vi "阈值图像分割.vi"() -> ()   [LabVIEW 2018]
doc: "This example shows how to open, read, and display an AVI file in NI Vision. The VI reads the frames per second property and plays the images back at the rate specified by the AVI file."
uses:
  <vilib>/Utility/file.llb/Read Delimited Spreadsheet (DBL).vi
  <vilib>/Utility/file.llb/Write Delimited Spreadsheet (I64).vi
  <vilib>/vision/NI_Vision_Development_Module.lvlib
panel:
  in  "清除叠加火焰":bool
  in  "保存":bool
  out "像素当量单位":string
  out "像素当量":string
  out "帧数据":T1
  in  "保存按钮":bool
  out "叠加像素源":u8[][](array[numeric])
  out "总像素":dbl
  in  "暂停按钮":bool
  out "火焰帧数":string
  out "叠加实际":string
  out "单帧实际":string
  out "叠加像素":string
  out "单帧像素":string
  out "导入像素当量":bool
  in  "单帧回看":bool
  out "叠加部分":string
  out "单帧部分":string
  in  "火焰详细参数":bool
  in  "返回主界面":bool
  out "a直方图":dynamicdata(graph) caption="A直方图"
  out "L直方图":dynamicdata(graph)
  in  "b":cluster{i32, i32}(slide)={-21, 6} scale=-100.0..100.0
  in  "a":cluster{i32, i32}(slide)={-21, -7} scale=-100.0..100.0
  in  "L":cluster{i32, i32}(slide)={81, 99} scale=0.0..100.0
  out "图形处理后":T2(plugin-control)
  out "单幅画面":T2(plugin-control) caption="单帧画面"
  in  "帧数计数":i32(slide) max=25 scale=0.0..25.0
  in  "Stop":bool
  out "Threshold Image":T2(plugin-control) caption="原图"
  out "叠加画面":T2(plugin-control)
  out "b直方图":dynamicdata(graph) caption="B直方图"
  # "基于Lab颜色空间的炮口火焰阈值分割"
  # "火焰参数"
  # "Lab颜色直方图&阈值选择"
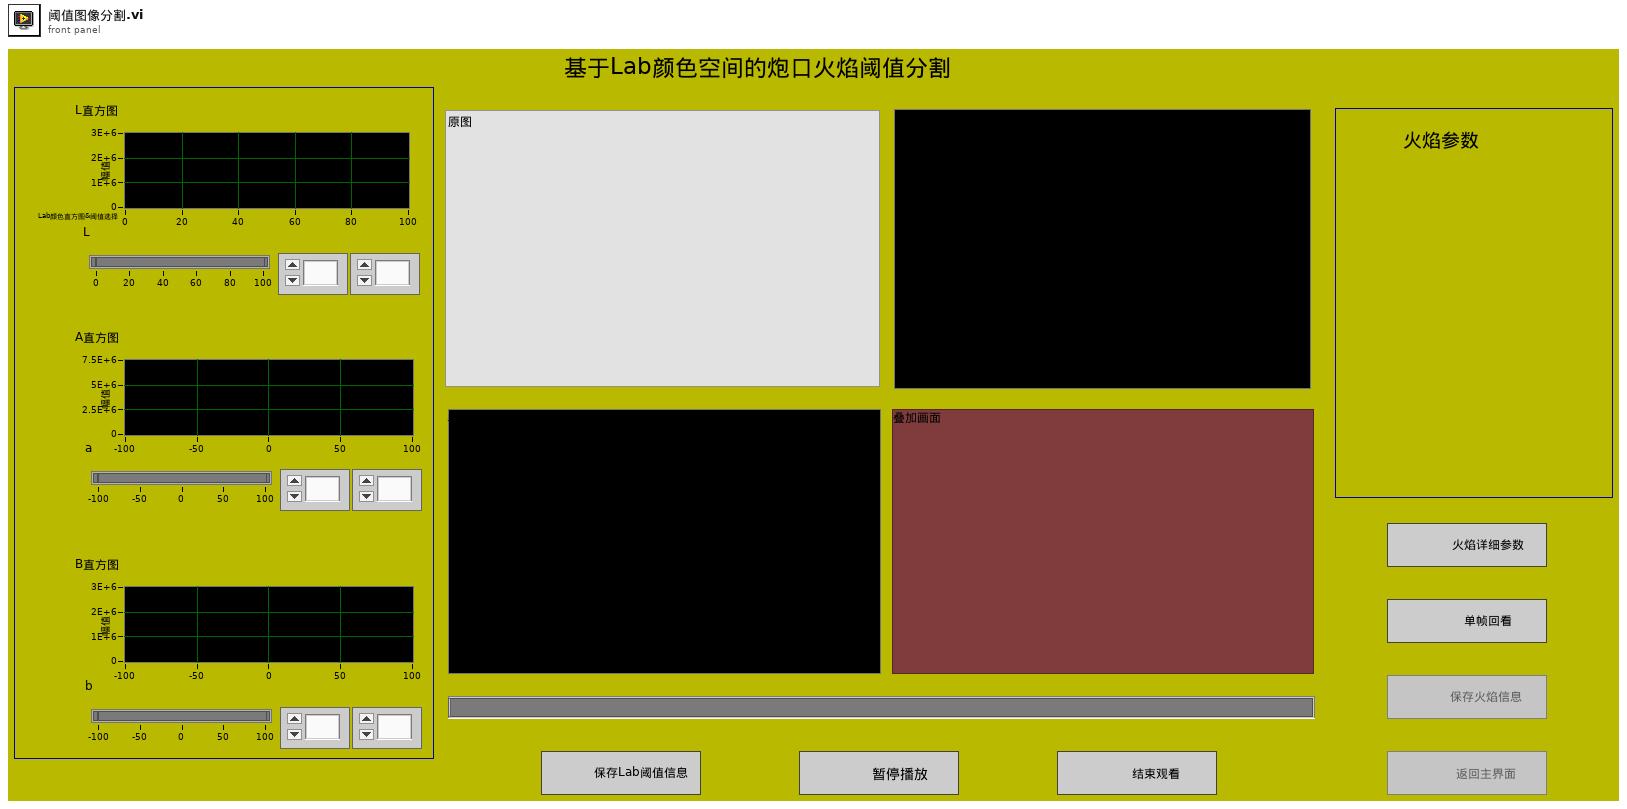
[diagram p1: front panel]
types:
  T1 = cluster{"Width":u32, "Height":u32, "Frames Per Second":u32, "Codec":string, "Has Data":bool}
  T2 = typedef "IMAQ Image.ctl" = refnum<image>
  T3 = enum8{"Enabled", "Disabled", "Disabled and Grayed Out"}
  T4 = typedef "Image Type" = u32
  T5 = enum32{"Invalid", "Standard", "Closed", "Hidden", "Minimized", "Maximized"}
  T6 = typedef "IMAQ AVI2 Refnum.ctl" = refnum<k20>
  T7 = cluster{"X Size":i32, "Y Size":i32, "% Tolerance":i32}
  T8 = typedef "ROI Descriptor" = cluster{"Global Rectangle":i32[], "Contours":cluster{"ID":enum32{"External", "Internal"}, "Type":u32, "Coordinates":i32[]}[]}
  T9 = cluster{"Area":dbl, "Number of Holes":dbl, "Bounding Rect":cluster{"Left":dbl, "Top":dbl, "Right":dbl, "Bottom":dbl}, "Center of Mass":cluster{"X":dbl, "Y":dbl}, "Orientation":dbl, "Dimensions":cluster{"Width":dbl, "Height":dbl}}[]
  T10 = cluster{"Particle Reports (Pixels)[0]":cluster{"Area":dbl, "Number of Holes":dbl, "Bounding Rect":cluster{"Left":dbl, "Top":dbl, "Right":dbl, "Bottom":dbl}, "Center of Mass":cluster{"X":dbl, "Y":dbl}, "Orientation":dbl, "Dimensions":cluster{"Width":dbl, "Height":dbl}}, "Particle Reports (Pixels)[1]":cluster{"Area":dbl, "Number of Holes":dbl, "Bounding Rect":cluster{"Left":dbl, "Top":dbl, "Right":dbl, "Bottom":dbl}, "Center of Mass":cluster{"X":dbl, "Y":dbl}, "Orientation":dbl, "Dimensions":cluster{"Width":dbl, "Height":dbl}}, "Particle Reports (Pixels)[2]":cluster{"Area":dbl, "Number of Holes":dbl, "Bounding Rect":cluster{"Left":dbl, "Top":dbl, "Right":dbl, "Bottom":dbl}, "Center of Mass":cluster{"X":dbl, "Y":dbl}, "Orientation":dbl, "Dimensions":cluster{"Width":dbl, "Height":dbl}}, "Particle Reports (Pixels)[3]":cluster{"Area":dbl, "Number of Holes":dbl, "Bounding Rect":cluster{"Left":dbl, "Top":dbl, "Right":dbl, "Bottom":dbl}, "Center of Mass":cluster{"X":dbl, "Y":dbl}, "Orientation":dbl, "Dimensions":cluster{"Width":dbl, "Height":dbl}}, "Particle Reports (Pixels)[4]":cluster{"Area":dbl, "Number of Holes":dbl, "Bounding Rect":cluster{"Left":dbl, "Top":dbl, "Right":dbl, "Bottom":dbl}, "Center of Mass":cluster{"X":dbl, "Y":dbl}, "Orientation":dbl, "Dimensions":cluster{"Width":dbl, "Height":dbl}}, "Particle Reports (Pixels)[5]":cluster{"Area":dbl, "Number of Holes":dbl, "Bounding Rect":cluster{"Left":dbl, "Top":dbl, "Right":dbl, "Bottom":dbl}, "Center of Mass":cluster{"X":dbl, "Y":dbl}, "Orientation":dbl, "Dimensions":cluster{"Width":dbl, "Height":dbl}}, "Particle Reports (Pixels)[6]":cluster{"Area":dbl, "Number of Holes":dbl, "Bounding Rect":cluster{"Left":dbl, "Top":dbl, "Right":dbl, "Bottom":dbl}, "Center of Mass":cluster{"X":dbl, "Y":dbl}, "Orientation":dbl, "Dimensions":cluster{"Width":dbl, "Height":dbl}}, "Particle Reports (Pixels)[7]":cluster{"Area":dbl, "Number of Holes":dbl, "Bounding Rect":cluster{"Left":dbl, "Top":dbl, "Right":dbl, "Bottom":dbl}, "Center of Mass":cluster{"X":dbl, "Y":dbl}, "Orientation":dbl, "Dimensions":cluster{"Width":dbl, "Height":dbl}}, "Particle Reports (Pixels)[8]":cluster{"Area":dbl, "Number of Holes":dbl, "Bounding Rect":cluster{"Left":dbl, "Top":dbl, "Right":dbl, "Bottom":dbl}, "Center of Mass":cluster{"X":dbl, "Y":dbl}, "Orientation":dbl, "Dimensions":cluster{"Width":dbl, "Height":dbl}}}
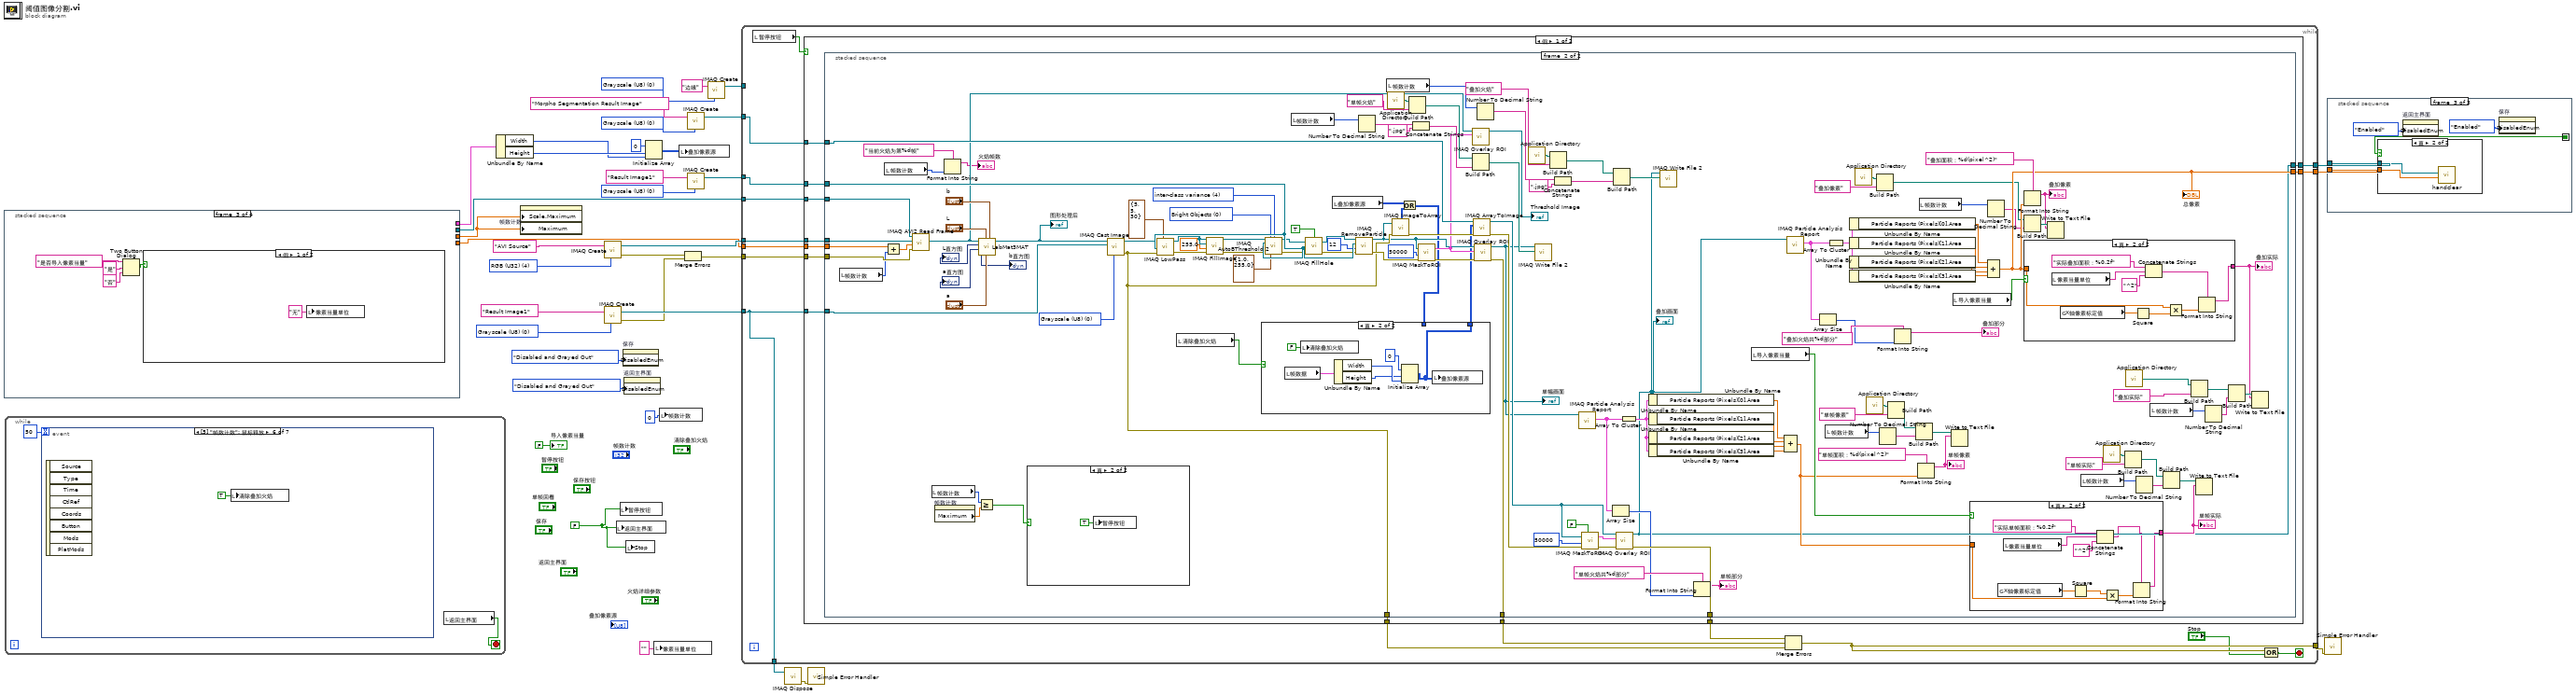
[diagram p0: block diagram]
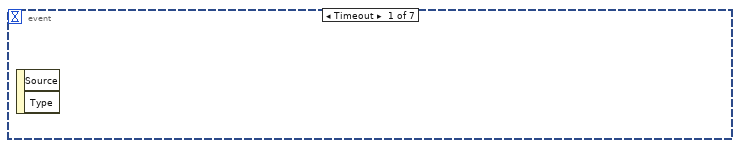
[diagram p2: hidden frame]
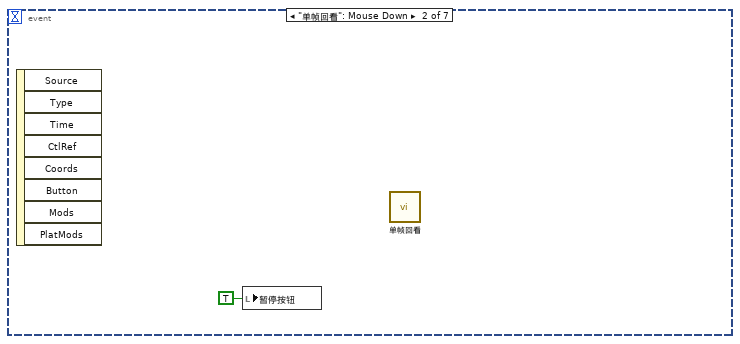
[diagram p3: hidden frame]
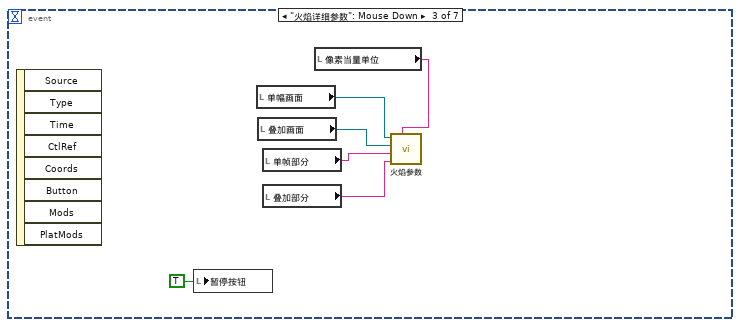
[diagram p4: hidden frame]
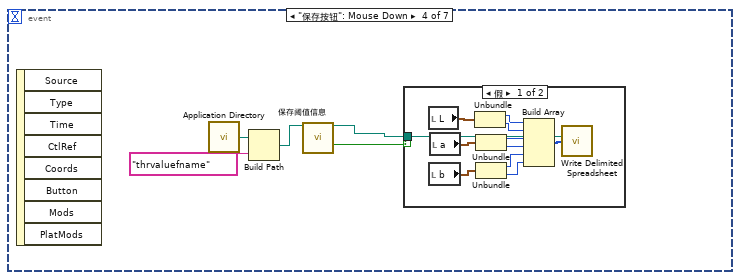
[diagram p5: hidden frame]
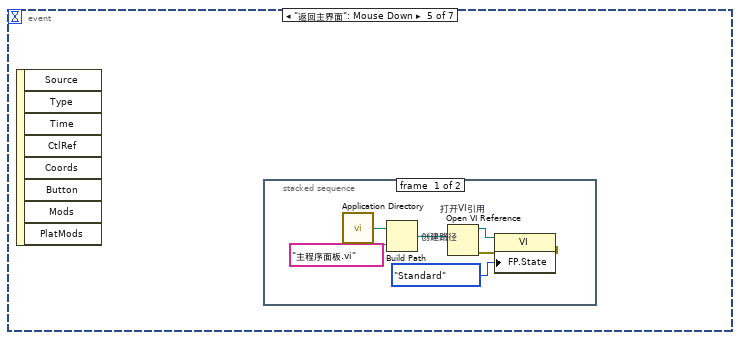
[diagram p7: hidden frame]
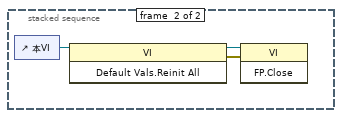
[diagram p8: hidden frame]
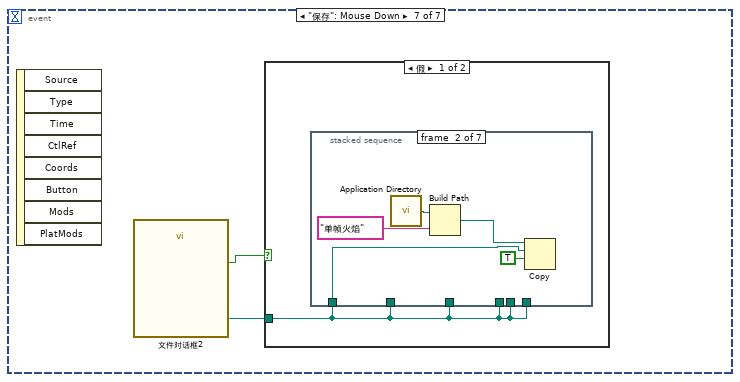
[diagram p9: hidden frame]
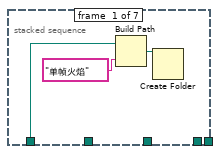
[diagram p10: hidden frame]
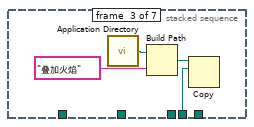
[diagram p11: hidden frame]
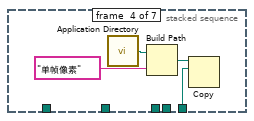
[diagram p12: hidden frame]
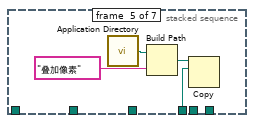
[diagram p13: hidden frame]
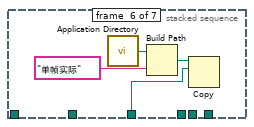
[diagram p14: hidden frame]
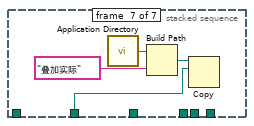
[diagram p15: hidden frame]
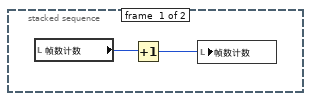
[diagram p17: hidden frame]
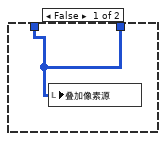
[diagram p18: hidden frame]
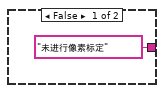
[diagram p20: hidden frame]
diagram:
  w3 = FALSE ("返回主界面")
  w13 = T4 0 items=["Grayscale (U8)", "Grayscale (I16)", "Grayscale (SGL)", "Complex (CSG)", "RGB (U32)", "HSL (U32)", "RGB (U64)", "Grayscale (U16)"] ("Image Type")
  w20 = T4 0 items=["Grayscale (U8)", "Grayscale (I16)", "Grayscale (SGL)", "Complex (CSG)", "RGB (U32)", "HSL (U32)", "RGB (U64)", "Grayscale (U16)"] ("Image Type")
  w27 = T4 0 items=["Grayscale (U8)", "Grayscale (I16)", "Grayscale (SGL)", "Complex (CSG)", "RGB (U32)", "HSL (U32)", "RGB (U64)", "Grayscale (U16)"] ("Image Type")
  w30 = T4 0 items=["Grayscale (U8)", "Grayscale (I16)", "Grayscale (SGL)", "Complex (CSG)", "RGB (U32)", "HSL (U32)", "RGB (U64)", "Grayscale (U16)"] ("Image Type")
  w32 = T4 4 items=["Grayscale (U8)", "Grayscale (I16)", "Grayscale (SGL)", "Complex (CSG)", "RGB (U32)", "HSL (U32)", "RGB (U64)", "Grayscale (U16)"] ("Image Type")
  n1 = stacked-sequence {
    tunnel: [w41 _ _ _] -> w16
    tunnel: [w42 _ _ _] -> w15
    tunnel: [w43 _ _ _] -> w9
    tunnel: [w40 _ _ _] -> w10
    frame #0 {
      n2 = control-ref of="本VI"() -> (w38:refnum<vi>)
      n3 = call "帧数选择.vi"() -> ("AVI Refnum"=w41:T6, "初始帧"=w40:dbl, "Frame Data"=w42:T1, "结束帧"=w43:dbl)  [unwired: 5 in, 1 out]
      "帧数据" <- w42
      n4 = property class="VI"(reference=w38, "FP.State"=T5."Hidden" ("前面板窗口:状态")) -> ()  [unwired: 1 in, 2 out]
    }
    frame #1 {
      n5 = while {
        stop <- w47 continue-if-true
        n6 = Current VI's Path() -> (path=w53:path)
        n7 = Strip Path(path=w53) -> (stripped path=w52:path)  [unwired: 1 out]
        n8 = Build Path(base path=w52, name or relative path="thrvaluefname") -> (appended path=w50:path)
        n9 = call "IMAQ Load Image Dialog"("Prompt"="请选择阈值文件，或点取消进入手动输入", "Pattern"="*.*", "Start Path"=w50) -> ("Cancelled?"=w46:bool, "Path"=w49:path)  [unwired: 6 in, 1 out]
        n10 = case shown="假" w46 {
          tunnel: w49 -> [w68 _]
          tunnel: [FALSE w69] -> w45
          frame False {
            n11 = call-poly <vilib>:"Read Delimited Spreadsheet.vi"("file path (dialog if empty)"=w68) -> ("all rows"=w67:dbl[][])  [unwired: 9 in, 5 out]
            n12 = Index Array(array=w67) -> (element #1=w66:dbl[], element #2=w59:dbl[], element #3=w58:dbl[])  [unwired: 6 in]
            n13 = Index Array(array=w66) -> (element #1=w64:dbl, element #2=w65:dbl)  [unwired: 2 in]
            n14 = Index Array(array=w59) -> (element #1=w62:dbl, element #2=w63:dbl)  [unwired: 2 in]
            n15 = Index Array(array=w58) -> (element #1=w60:dbl, element #2=w61:dbl)  [unwired: 2 in]
            n16 = Bundle("Numeric"=w64, "Numeric"=w65) -> (w57:cluster{"Numeric":dbl, "Numeric":dbl})  [unwired: 1 in]
            n17 = Bundle("Numeric"=w62, "Numeric"=w63) -> (w56:cluster{"Numeric":dbl, "Numeric":dbl})  [unwired: 1 in]
            n18 = Bundle("Numeric"=w60, "Numeric"=w61) -> (w55:cluster{"Numeric":dbl, "Numeric":dbl})  [unwired: 1 in]
            n19 = local write "a"(w56) -> ()
            n20 = local write "L"(w57) -> ()
            n21 = local write "b"(w55) -> ()
          }
          frame True {
            n22 = Two Button Dialog(message="请输入阈值 ，否者程序运行有误，手动输入，还是从文件读取", 1:"手动输入" ("Center Button Text (\"No\")"), 2:"从文件读入" ("Left Button Text (\"Yes\")")) -> (T button?=w70:bool)
            n23 = case shown="真" w70 {
              selector: w70 -> [_ w78]
              tunnel: [FALSE w78] -> w69
              frame False {
                n24 = call "thrhand.vi"() -> ("b"=w74:cluster{"bmin":dbl, "bmax":dbl}, "a"=w75:cluster{"amin":dbl, "amax":dbl}, "L"=w76:cluster{"Lmin":dbl, "Lmax":dbl})
                n25 = local write "a"(w75) -> ()
                n26 = local write "L"(w76) -> ()
                n27 = local write "b"(w74) -> ()
              }
              frame True {
              }
            }
          }
        }
        n28 = And(x=w45, y=w46) -> (x .and. y?=w47:bool)
      }
    }
    frame #2 {
      n29 = Two Button Dialog(message="是否导入像素当量" ("消息"), 1:"否" ("F按钮名称（“取消”）"), 2:"是" ("T按钮名称（“确定”）")) -> (T button?=w82:bool)
      n30 = case shown="假" w82 {
        frame False {
          n31 = local write "像素当量单位"("无" ("像素当量单位")) -> ()
        }
        frame True {
          n32 = stacked-sequence {
            frame #0 {
              n33 = local write "导入像素当量"(TRUE ("导入像素当量")) -> ()
              n34 = call "文件对话框"("default name"="请选择像素当量") -> ("selected path"=w88:path)  [unwired: 11 in, 3 out]
              n35 = Read from Text File(file (use dialog)=w88) -> (text=w87:string)  [unwired: 3 in, 3 out]
              "像素当量" <- w87
              n36 = Fract/Exp String To Number(string=w87) -> (number=w86:dbl)  [unwired: 3 in, 1 out]
              n37 = global write "全局变量.vi" "X轴像素标定值"(w86) -> ()
              n38 = global write "全局变量.vi" "Y轴像素标定值"(w86) -> ()
            }
            frame #1 {
              n39 = invoke on="像素当量" class="Str" method="Get Nth Line"("index"=u32 2 ("行索引")) -> (error out=w91:errorcluster, "text"=w90:string)  [unwired: 6 in, 5 out]
              n40 = case shown="错误" w91 {
                selector: w91 -> [_ w95]
                tunnel: w90 -> [w92 _]
                frame No Error {
                  "像素当量单位" <- w92
                }
                frame Error {
                  n41 = local write "像素当量单位"("无" ("像素当量单位")) -> ()
                  n42 = One Button Dialog(message="导入像素当量单位时出错，\n请检查导入文件是否正确。" ("消息")) -> ()  [unwired: 1 in, 1 out]
                  n43 = call <vilib>:"Simple Error Handler.vi"("error in (no error)"=w95) -> ()  [unwired: 4 in, 5 out]
                }
              }
            }
          }
        }
      }
    }
    frame #3 {
      n44 = flat-sequence {
        frame #0 {
          n45 = control-ref of="本VI"() -> (w97:refnum<vi>)
          n46 = property class="VI"(reference=w97, "FP.State"=T5."Standard" ("前面板窗口:状态")) -> ()  [unwired: 1 in, 2 out]
        }
        frame #1 {
          n47 = Wait (ms)(milliseconds to wait=u32 200 ("等待时间（毫秒）")) -> ()  [unwired: 1 out]
        }
      }
    }
  }
  n48 = while {
    stop <- w99 stop-if-true
    n49 = event "事件结构" shown="[5] \"帧数计数\": 鼠标释放" {
      selector: _ -> [_ _ _ _ _ _ _]
      dyn-events: _ -> [_ _ _ _ _ _ _]
      timeout: 50 -> [_ _ _ _ _ _ _]
      event Timeout {
        n50 = event-data() -> ()  [unwired: 1 in, 2 out]
      }
      event "单帧回看": Mouse Down {
        n51 = event-data() -> ()  [unwired: 1 in, 8 out]
        n52 = local write "暂停按钮"(TRUE ("暂停按钮")) -> ()
        n53 = call "单帧回看.vi"() -> ()  [unwired: 28 in]
      }
      event "火焰详细参数": Mouse Down {
        n54 = event-data() -> ()  [unwired: 1 in, 8 out]
        n55 = local write "暂停按钮"(TRUE ("暂停按钮")) -> ()
        n56 = local read "单幅画面"() -> (w105:T2)
        n57 = local read "叠加画面"() -> (w104:T2)
        n58 = local read "单帧部分"() -> (w107:string)
        n59 = local read "叠加部分"() -> (w106:string)
        n60 = local read "像素当量单位"() -> (w102:string)
        n61 = call "火焰参数.vi"("像素当量单位"=w102, 8:w106, 9:w107, "Image 2"=w104, "Image"=w105) -> ()  [unwired: 7 in]
      }
      event "保存按钮": Mouse Down {
        n62 = event-data() -> ()  [unwired: 1 in, 8 out]
        n63 = call <vilib>:"Application Directory.vi"() -> ("Application Directory"=w110:path)
        n64 = Build Path(base path=w110, name or relative path="thrvaluefname") -> (appended path=w109:path)
        n65 = call "保存阈值信息"("start path"=w109) -> ("selected path"=w112:path, "cancelled"=w108:bool)  [unwired: 11 in, 2 out]
        n66 = case shown="假" w108 {
          tunnel: w112 -> [w123 _]
          frame False {
            n67 = local read "L"() -> (w113:cluster{i32, i32})
            n68 = local read "b"() -> (w115:cluster{i32, i32})
            n69 = local read "a"() -> (w114:cluster{i32, i32})
            n70 = Unbundle(w113) -> (w116:i32, w117:i32)
            n71 = Unbundle(w114) -> (w118:i32, w119:i32)
            n72 = Unbundle(w115) -> (w120:i32, w121:i32)
            n73 = Build Array(w116, w117, w118, w119, w120, w121) -> (w122:i32[])
            n74 = call-poly <vilib>:"Write Delimited Spreadsheet.vi"("file path (dialog if empty)"=w123, "1D data"=w122) -> ()  [unwired: 12 in, 2 out]
          }
          frame True {
          }
        }
      }
      event "返回主界面": Mouse Down {
        n75 = event-data() -> ()  [unwired: 1 in, 8 out]
        n76 = stacked-sequence {
          frame #0 {
            n77 = call <vilib>:"Application Directory.vi"() -> ("Application Directory"=w124:path)
            n78 = Build Path "创建路径"(base path=w124, name or relative path="主程序面板.vi" ("名称或相对路径")) -> (appended path=w129:path)
            n79 = Open VI Reference "打开VI引用"(vi path=w129) -> (vi reference=w128:refnum<vi>, error out=w127:errorcluster)  [unwired: 5 in]
            n80 = property class="VI"(reference=w128, error in=w127, "FP.State"=T5."Standard" ("前面板窗口:状态")) -> ()  [unwired: 2 out]
          }
          frame #1 {
            n81 = control-ref of="本VI"() -> (w130:refnum<vi>)
            n82 = invoke class="VI" method="Default Vals.Reinit All"(reference=w130) -> (reference out=w131:refnum<vi>, error out=w132:errorcluster)  [unwired: 2 in, 1 out]
            n83 = invoke class="VI" method="FP.Close"(reference=w131, error in=w132) -> ()  [unwired: 1 in, 3 out]
          }
        }
      }
      event "帧数计数": Mouse Up {
        n84 = event-data() -> ()  [unwired: 1 in, 8 out]
        n85 = local write "清除叠加火焰"(TRUE ("清除叠加火焰")) -> ()
      }
      event "保存": Mouse Down {
        n86 = event-data() -> ()  [unwired: 1 in, 8 out]
        n87 = call "文件对话框2"() -> ("selected path"=w134:path, "cancelled"=w135:bool)  [unwired: 12 in, 2 out]
        n88 = case shown="假" w135 {
          tunnel: w134 -> [w136 _]
          frame False {
            n89 = stacked-sequence {
              tunnel: w136 -> [w137 w141 _ _ _ _ _]
              tunnel: w136 -> [_ _ w146 _ _ _ _]
              tunnel: w136 -> [_ _ _ w150 _ _ _]
              tunnel: w136 -> [_ _ _ _ w154 _ _]
              tunnel: w136 -> [_ _ _ _ _ w158 _]
              tunnel: w136 -> [_ _ _ _ _ _ w161]
              frame #0 {
                n90 = Build Path(base path=w137, name or relative path="单帧火焰" ("名称或相对路径")) -> (appended path=w139:path)
                n91 = Create Folder(path (use dialog)=w139) -> ()  [unwired: 2 in, 3 out]
              }
              frame #1 {
                n92 = call <vilib>:"Application Directory.vi"() -> ("Application Directory"=w144:path)
                n93 = Build Path(base path=w144, name or relative path="单帧火焰" ("名称或相对路径")) -> (appended path=w142:path)
                n94 = Copy(9:TRUE ("覆盖(F)"), 10:w141, 11:w142) -> ()  [unwired: 2 in, 3 out]
              }
              frame #2 {
                n95 = call <vilib>:"Application Directory.vi"() -> ("Application Directory"=w147:path)
                n96 = Build Path(base path=w147, name or relative path="叠加火焰" ("名称或相对路径")) -> (appended path=w148:path)
                n97 = Copy(10:w146, 11:w148) -> ()  [unwired: 3 in, 3 out]
              }
              frame #3 {
                n98 = call <vilib>:"Application Directory.vi"() -> ("Application Directory"=w151:path)
                n99 = Build Path(base path=w151, name or relative path="单帧像素" ("名称或相对路径")) -> (appended path=w152:path)
                n100 = Copy(10:w150, 11:w152) -> ()  [unwired: 3 in, 3 out]
              }
              frame #4 {
                n101 = call <vilib>:"Application Directory.vi"() -> ("Application Directory"=w155:path)
                n102 = Build Path(base path=w155, name or relative path="叠加像素" ("名称或相对路径")) -> (appended path=w156:path)
                n103 = Copy(10:w154, 11:w156) -> ()  [unwired: 3 in, 3 out]
              }
              frame #5 {
                n104 = call <vilib>:"Application Directory.vi"() -> ("Application Directory"=w159:path)
                n105 = Build Path(base path=w159, name or relative path="单帧实际" ("名称或相对路径")) -> (appended path=w160:path)
                n106 = Copy(10:w158, 11:w160) -> ()  [unwired: 3 in, 3 out]
              }
              frame #6 {
                n107 = call <vilib>:"Application Directory.vi"() -> ("Application Directory"=w163:path)
                n108 = Build Path(base path=w163, name or relative path="叠加实际" ("名称或相对路径")) -> (appended path=w164:path)
                n109 = Copy(10:w161, 11:w164) -> ()  [unwired: 3 in, 3 out]
              }
            }
          }
          frame True {
          }
        }
      }
    }
    n110 = local read "返回主界面"() -> (w99:bool)
  }
  n111 = Unbundle By Name(w15) -> ("Width"=w23:u32, "Height"=w24:u32)
  n112 = property on="帧数计数" class="Slide (严格)"("Scale.Maximum"=w9, "Maximum"=w9) -> ()  [unwired: 2 in, 2 out]
  n113 = call "IMAQ Create"("Image Name"="AVI Source", "Image Type"=w32) -> ("New Image"=w33:T2, "error out"=w36:errorcluster)  [unwired: 2 in, 1 out]
  n114 = call "IMAQ Create"("Image Name"="Result Image1", "Image Type"=w20) -> ("New Image"=w19:T2, "error out"=w17:errorcluster)  [unwired: 2 in, 1 out]
  n115 = local write "返回主界面"(w3) -> ()
  n116 = local write "暂停按钮"(w3) -> ()
  n117 = property on="保存" class="Bool (严格)"("DisabledEnum"=T3."Disabled and Grayed Out" ("禁用")) -> ()  [unwired: 2 in, 2 out]
  n118 = property on="返回主界面" class="Bool (严格)"("DisabledEnum"=T3."Disabled and Grayed Out" ("禁用")) -> ()  [unwired: 2 in, 2 out]
  n119 = local write "Stop"(w3) -> ()
  n120 = Initialize Array(u8 0 ("元素"), w24, w23) -> (w4:u8[][])
  n121 = local write "像素当量单位"("" ("像素当量单位")) -> ()
  n122 = local write "帧数计数"(0 ("数值输入控件")) -> ()
  n123 = local write "叠加像素源"(w4) -> ()
  n124 = Merge Errors(w36, w17) -> (w35:errorcluster)
  n125 = call "IMAQ Create"("Image Name"="Morpho Segmentation Result Image", "Image Type"=w27) -> ("New Image"=w26:T2)  [unwired: 2 in, 2 out]
  n126 = call "IMAQ Create"("Image Name"="Result Image1", "Image Type"=w30) -> ("New Image"=w29:T2)  [unwired: 2 in, 2 out]
  n127 = call "IMAQ Create"("Image Name"="边缘", "Image Type"=w13) -> ("New Image"=w11:T2)  [unwired: 2 in, 2 out]
  n128 = while {
    tunnel: [w178] -> w5
    tunnel: w35 -> [w174]
    tunnel: w16 -> [w176]
    tunnel: w33 -> [w175]
    tunnel: [w166] -> w28
    tunnel: w29 -> [w177]
    tunnel: w26 -> [w179]
    tunnel: w19 -> [w173]
    tunnel: [w173] -> w18
    tunnel: [w167] -> w14
    tunnel: w11 -> [_]
    tunnel: w10 -> [w168]
    stop <- w180 stop-if-true
    n129 = local read "暂停按钮"() -> (w165:bool)
    n130 = case shown="假" w165 {
      tunnel: w179 -> [w192 _]
      tunnel: w177 -> [w191 w365]
      tunnel: w176 -> [w190 w360]
      tunnel: w175 -> [w189 w361]
      tunnel: w174 -> [w188 _]
      tunnel: w173 -> [w187 w379]
      tunnel: [w186 _] -> w171
      tunnel: [w185 _] -> w170
      tunnel: [w184 _] -> w169
      tunnel: w168 -> [w183 w364]
      tunnel: [w182 w391] -> w167
      tunnel: [w181 w390] -> w166
      frame False {
        n131 = stacked-sequence {
          tunnel: w192 -> [_ w325]
          tunnel: w191 -> [_ w324]
          tunnel: w190 -> [_ w323]
          tunnel: w189 -> [_ w322]
          tunnel: w188 -> [_ w321]
          tunnel: w187 -> [_ w320]
          tunnel: [_ w296] -> w186
          tunnel: [_ w295] -> w185
          tunnel: [_ w292] -> w184
          tunnel: w183 -> [_ w270]
          tunnel: [_ w253] -> w182
          tunnel: [_ w204] -> w181
          frame #0 {
            n132 = local read "帧数计数"() -> (w194:i32)
            n133 = Increment(x=w194) -> (x+1=w193:i32)
            n134 = local write "帧数计数"(w193) -> ()
          }
          frame #1 {
            w312 = u32 0 items=["Bright Objects", "Dark Objects"] ("Look For (Bright Objects)")
            w315 = 4 items=["clustering", "entropy", "metric", "moments", "inter-class variance"] ("Method")
            w316 = T4 0 items=["Grayscale (U8)", "Grayscale (I16)", "Grayscale (SGL)", "Complex (CSG)", "RGB (U32)", "HSL (U32)", "RGB (U64)", "Grayscale (U16)"] ("Image Type")
            n135 = local read "帧数计数"() -> (w203:i32)
            n136 = local read "帧数计数"() -> (w202:i32)
            n137 = Add(x=w270, y=w203) -> (x+y=w269:dbl)
            n138 = call "IMAQ AVI2 Read Frame"("error in (no error)"=w321, "Frame Number"=w269, "Image"=w322, "AVI Refnum"=w323) -> ("Image Out"=w268:T2)  [unwired: 7 out]
            n139 = local read "帧数计数"() -> (w201:i32)
            n140 = property on="帧数计数" class="Slide (严格)"() -> ("Maximum"=w200:dbl)  [unwired: 2 in, 2 out]
            n141 = Format Into String(format string="当前火焰为第%d帧" ("格式字符串"), w202) -> (resulting string=→"火焰帧数":string)  [unwired: 2 in, 1 out]
            n142 = Greater Or Equal?(x=w201, y=w200) -> (x >= y?=w199:bool)
            n143 = call "LabMat3MAT.vi"("b"="b", "a"="a", "L"="L", "Image"=w268) -> ("Image  output"=w283:T2, "Histogram 3"=→"b直方图":dynamicdata, "Histogram 2"=→"a直方图":dynamicdata, "Histogram"=→"L直方图":dynamicdata)  [unwired: 3 in, 1 out]
            "图形处理后" <- w283
            n144 = case shown="真" w199 {
              frame False {
              }
              frame True {
                n145 = local write "暂停按钮"(TRUE ("暂停按钮")) -> ()
              }
            }
            n146 = call "IMAQ Cast Image"("Image Type"=w316, "Image Dst"=w320, "Image Src"=w283) -> ("error out"=w295:errorcluster, "Image Dst Out"=w284:T2)  [unwired: 7 in]
            n147 = call "IMAQ LowPass"("Image Src"=w284, "Size & Tolerance"=T7 {"X Size"=5, "Y Size"=5, "% Tolerance"=30}, "Image Dst"=w324, "error in (no error)"=w295) -> ("Image Dst Out"=w299:T2, "error out"=w303:errorcluster)  [unwired: 3 in]
            n148 = local read "清除叠加火焰"() -> (w197:bool)
            n149 = call "IMAQ FillImage"("error in (no error)"=w303, "Pixel Value (U8, U16, I16, Float)"=sgl 255.0, "Image Mask"=w299, "Image"=w299) -> ("error out"=w302:errorcluster, "Image Out"=w298:T2)  [unwired: 6 in]
            n150 = call "IMAQ AutoBThreshold 2"("Image Src"=w298, "Look For (Bright Objects)"=w312, "Method (clustering)"=w315, "Image Dst"=w324, "error in (no error)"=w302, "Threshold Limits"=cluster{"Lower value":sgl, "Upper value":sgl} {"Lower value"=1.0, "Upper value"=255.0}) -> ("Image Dst Out"=w301:T2, "error out"=w314:errorcluster)  [unwired: 2 in, 6 out]
            n151 = local read "帧数计数"() -> (w221:i32)
            n152 = call "IMAQ FillHole"("error in (no error)"=w314, "Image Dst"=w324, "Image Src"=w301, "Connectivity 4/8 (8)"=TRUE) -> ("error out"=w310:errorcluster, "Image Dst Out"=w300:T2)  [unwired: 2 in]
            n153 = local read "叠加像素源"() -> (w198:u8[][])
            n154 = call "IMAQ RemoveParticle"("error in (no error)"=w310, "Number of Erosion"=12, "Image Dst"=w324, "Image Src"=w300) -> ("error out"=w308:errorcluster, "Image Dst Out"=w273:T2)  [unwired: 6 in]
            n155 = Number To Decimal String(number=w221) -> (decimal integer string=w217:string)  [unwired: 1 in]
            n156 = local read "帧数计数"() -> (w205:i32)
            n157 = call <vilib>:"Application Directory.vi"() -> ("Application Directory"=w218:path)
            n158 = call "IMAQ ImageToArray"("error in (no error)"=w295, "Image"=w273) -> ("error out"=w294:errorcluster, "Image Pixels (U8)"=w297:u8[][])  [unwired: 2 in, 3 out]
            n159 = Or(x=w198, y=w297) -> (x .or. y?=w196:u8[][])
            n160 = case shown="真" w197 {
              tunnel: w196 -> [w326 _]
              tunnel: [w326 w327] -> w195
              frame False {
                n161 = local write "叠加像素源"(w326) -> ()
              }
              frame True {
                n162 = local read "帧数据"() -> (w330:T1)
                n163 = local write "清除叠加火焰"(FALSE ("清除叠加火焰")) -> ()
                n164 = Unbundle By Name(w330) -> ("Width"=w332:u32, "Height"=w331:u32)
                n165 = Initialize Array(0, w331, w332) -> (w327:i32[][])
                n166 = local write "叠加像素源"(w327) -> ()
              }
            }
            n167 = Build Path(base path=w218, name or relative path="单帧火焰" ("名称或相对路径")) -> (appended path=w220:path)
            n168 = Concatenate Strings(w217, ".jpg" ("字符串")) -> (w215:string)
            n169 = call "IMAQ MaskToROI"("Image"=w273, "Max number of vectors in ROI"=50000, "error in (no error)"=w308) -> ("ROI Descriptor"=w272:T8, "error out"=w307:errorcluster)  [unwired: 4 in, 1 out]
            n170 = call "IMAQ Overlay ROI"("ROI Descriptor"=w272, "Image"=w268) -> ("Image Out"=→"Threshold Image":T2)  [unwired: 8 in, 1 out]
            n171 = Build Path(base path=w220, name or relative path=w215) -> (appended path=w214:path)
            n172 = call "IMAQ ArrayToImage"("error in (no error)"=w294, "Image Pixels (U8)"=w195, "Image"=w325) -> ("error out"=w293:errorcluster, "Image Out"=w291:T2)  [unwired: 7 in]
            n173 = call "IMAQ Overlay ROI"("error in (no error)"=w307, "ROI Descriptor"=w272, "Image"=w273) -> ("error out"=w296:errorcluster, "Image Out"=w213:T2)  [unwired: 7 in]
            "单幅画面" <- w213
            n174 = Number To Decimal String(number=w205) -> (decimal integer string=w209:string)  [unwired: 1 in]
            n175 = call <vilib>:"Application Directory.vi"() -> ("Application Directory"=w208:path)
            n176 = call-poly "IMAQ Write File 2"("File Path"=w214, "Image"=w213) -> ()  [unwired: 8 in, 2 out]
            n177 = Build Path(base path=w208, name or relative path="叠加火焰" ("名称或相对路径")) -> (appended path=w206:path)
            n178 = Concatenate Strings(w209, ".jpg" ("字符串")) -> (w211:string)
            n179 = call "IMAQ Particle Analysis Report"("Image"=w213) -> ("Particle Reports (Pixels)"=w279:T9)  [unwired: 5 in, 5 out]
            n180 = call "IMAQ MaskToROI"("External edges only (T)"=FALSE, "Image"=w291, "Max number of vectors in ROI"=50000, "error in (no error)"=w293) -> ("ROI Descriptor"=w319:T8, "error out"=w318:errorcluster)  [unwired: 3 in, 1 out]
            n181 = Array Size(array=w279) -> (size(s)=w275:i32)
            n182 = Build Path(base path=w206, name or relative path=w211) -> (appended path=w212:path)
            n183 = call "IMAQ Overlay ROI"("error in (no error)"=w318, "ROI Descriptor"=w319, "Image"=w291) -> ("error out"=w292:errorcluster, "Image Out"=w204:T2)  [unwired: 7 in]
            "叠加画面" <- w204
            n184 = Array To Cluster(array=w279) -> (cluster=w267:T10)
            n185 = Unbundle By Name(w267) -> ("Particle Reports (Pixels)[0].Area"=w266:dbl)
            n186 = Unbundle By Name(w267) -> ("Particle Reports (Pixels)[1].Area"=w265:dbl)
            n187 = Unbundle By Name(w267) -> ("Particle Reports (Pixels)[2].Area"=w264:dbl)
            n188 = Unbundle By Name(w267) -> ("Particle Reports (Pixels)[3].Area"=w263:dbl)
            n189 = call-poly "IMAQ Write File 2"("File Path"=w212, "Image"=w204) -> ()  [unwired: 8 in, 2 out]
            n190 = Format Into String(format string="单帧火焰共%d部分" ("初始字符串"), w275) -> (resulting string=→"单帧部分":string)  [unwired: 2 in, 1 out]
            n191 = local read "导入像素当量"() -> (w255:bool)
            n192 = Compound Arithmetic op=ADD(w266, w265, w264, w263) -> (w254:dbl)
            n193 = call "IMAQ Particle Analysis Report"("Image"=w204) -> ("Particle Reports (Pixels)"=w276:T9)  [unwired: 5 in, 5 out]
            n194 = Array Size(array=w276) -> (size(s)=w274:i32)
            n195 = local read "帧数计数"() -> (w225:i32)
            n196 = Array To Cluster(array=w276) -> (cluster=w262:T10)
            n197 = Unbundle By Name(w262) -> ("Particle Reports (Pixels)[0].Area"=w261:dbl)
            n198 = Unbundle By Name(w262) -> ("Particle Reports (Pixels)[1].Area"=w260:dbl)
            n199 = Unbundle By Name(w262) -> ("Particle Reports (Pixels)[2].Area"=w259:dbl)
            n200 = Unbundle By Name(w262) -> ("Particle Reports (Pixels)[3].Area"=w258:dbl)
            n201 = call <vilib>:"Application Directory.vi"() -> ("Application Directory"=w240:path)
            n202 = call <vilib>:"Application Directory.vi"() -> ("Application Directory"=w223:path)
            n203 = Build Path(base path=w240, name or relative path="叠加像素" ("名称或相对路径")) -> (appended path=w239:path)
            n204 = Number To Decimal String(number=w225) -> (decimal integer string=w226:string)  [unwired: 1 in]
            n205 = Build Path(base path=w223, name or relative path="单帧像素" ("名称或相对路径")) -> (appended path=w224:path)
            n206 = Format Into String(format string="叠加火焰共%d部分" ("初始字符串"), w274) -> (resulting string=→"叠加部分":string)  [unwired: 2 in, 1 out]
            n207 = Build Path(base path=w224, name or relative path=w226) -> (appended path=w227:path)
            n208 = Format Into String(format string="单帧面积：%d(pixel^2)" ("格式字符串"), w254) -> (resulting string=w222:string)  [unwired: 2 in, 1 out]
            "单帧像素" <- w222
            n209 = local read "帧数计数"() -> (w237:i32)
            n210 = Write to Text File(file (use dialog)=w227, text=w222) -> ()  [unwired: 2 in, 3 out]
            n211 = local read "导入像素当量"() -> (w252:bool)
            n212 = case shown="真" w255 {
              tunnel: w254 -> [_ w351]
              tunnel: ["未进行像素标定" w349] -> w229
              frame False {
              }
              frame True {
                n213 = global read "全局变量.vi" "X轴像素标定值"() -> (w353:dbl)
                n214 = local read "像素当量单位"() -> (w348:string)
                n215 = Square(x=w353) -> (x^2=w352:dbl)
                n216 = Concatenate Strings("实际单帧面积：%0.2f" ("格式字符串"), w348, "^2" ("字符串")) -> (w345:string)
                n217 = Multiply(x=w352, y=w351) -> (x*y=w350:dbl)
                n218 = Format Into String(format string=w345, w350) -> (resulting string=w349:string)  [unwired: 2 in, 1 out]
              }
            }
            "单帧实际" <- w229
            n219 = Number To Decimal String(number=w237) -> (decimal integer string=w238:string)  [unwired: 1 in]
            n220 = Compound Arithmetic op=ADD(w261, w260, w259, w258) -> (w253:dbl)
            "总像素" <- w253
            n221 = Format Into String(format string="叠加面积：%d(pixel^2)" ("格式字符串"), w253) -> (resulting string=w236:string)  [unwired: 2 in, 1 out]
            "叠加像素" <- w236
            n222 = Build Path(base path=w239, name or relative path=w238) -> (appended path=w242:path)
            n223 = case shown="真" w252 {
              tunnel: ["未进行像素标定" w341] -> w243
              tunnel: w253 -> [_ w339]
              frame False {
              }
              frame True {
                n224 = local read "像素当量单位"() -> (w335:string)
                n225 = global read "全局变量.vi" "X轴像素标定值"() -> (w343:dbl)
                n226 = Square(x=w343) -> (x^2=w340:dbl)
                n227 = Concatenate Strings("实际叠加面积：%0.2f" ("格式字符串"), w335, "^2" ("字符串")) -> (w336:string)
                n228 = Multiply(x=w339, y=w340) -> (x*y=w342:dbl)
                n229 = Format Into String(format string=w336, w342) -> (resulting string=w341:string)  [unwired: 2 in, 1 out]
              }
            }
            "叠加实际" <- w243
            n230 = Write to Text File(file (use dialog)=w242, text=w236) -> ()  [unwired: 2 in, 3 out]
            n231 = local read "帧数计数"() -> (w233:i32)
            n232 = call <vilib>:"Application Directory.vi"() -> ("Application Directory"=w235:path)
            n233 = Build Path(base path=w235, name or relative path="单帧实际" ("名称或相对路径")) -> (appended path=w234:path)
            n234 = call <vilib>:"Application Directory.vi"() -> ("Application Directory"=w249:path)
            n235 = Number To Decimal String(number=w233) -> (decimal integer string=w232:string)  [unwired: 1 in]
            n236 = local read "帧数计数"() -> (w246:i32)
            n237 = Build Path(base path=w234, name or relative path=w232) -> (appended path=w231:path)
            n238 = Build Path(base path=w249, name or relative path="叠加实际" ("名称或相对路径")) -> (appended path=w247:path)
            n239 = Write to Text File(file (use dialog)=w231, text=w229) -> ()  [unwired: 2 in, 3 out]
            n240 = Number To Decimal String(number=w246) -> (decimal integer string=w245:string)  [unwired: 1 in]
            n241 = Build Path(base path=w247, name or relative path=w245) -> (appended path=w244:path)
            n242 = Write to Text File(file (use dialog)=w244, text=w243) -> ()  [unwired: 2 in, 3 out]
          }
        }
      }
      frame True {
        w374 = u32 0 items=["Bright Objects", "Dark Objects"] ("Look For (Bright Objects)")
        w373 = 4 items=["clustering", "entropy", "metric", "moments", "inter-class variance"] ("Method")
        w381 = T4 0 items=["Grayscale (U8)", "Grayscale (I16)", "Grayscale (SGL)", "Complex (CSG)", "RGB (U32)", "HSL (U32)", "RGB (U64)", "Grayscale (U16)"] ("Image Type")
        n243 = local read "帧数计数"() -> (w363:i32)
        n244 = Add(x=w364, y=w363) -> (x+y=w362:dbl)
        n245 = call "IMAQ AVI2 Read Frame"("Frame Number"=w362, "Image"=w361, "AVI Refnum"=w360) -> ("Image Out"=w357:T2)  [unwired: 1 in, 7 out]
        n246 = local read "L"() -> (w384:cluster{i32, i32})
        n247 = local read "a"() -> (w385:cluster{i32, i32})
        n248 = local read "b"() -> (w386:cluster{i32, i32})
        n249 = call "LabMat3MAT.vi"("b"=w386, "a"=w385, "L"=w384, "Image"=w357) -> ("Image  output"=w380:T2, "Histogram 3"=w389:dynamicdata, "Histogram 2"=w388:dynamicdata, "Histogram"=w387:dynamicdata)  [unwired: 3 in, 1 out]
        n250 = local write "图形处理后"(w380) -> ()
        n251 = local write "a直方图"(w388) -> ()
        n252 = local write "L直方图"(w387) -> ()
        n253 = local write "b直方图"(w389) -> ()
        n254 = call "IMAQ Cast Image"("Image Type"=w381, "Image Dst"=w379, "Image Src"=w380) -> ("error out"=w376:errorcluster, "Image Dst Out"=w383:T2)  [unwired: 7 in]
        n255 = call "IMAQ LowPass"("Image Src"=w383, "Size & Tolerance"=T7 {"X Size"=5, "Y Size"=5, "% Tolerance"=30}, "Image Dst"=w365, "error in (no error)"=w376) -> ("Image Dst Out"=w377:T2, "error out"=w375:errorcluster)  [unwired: 3 in]
        n256 = call "IMAQ FillImage"("error in (no error)"=w375, "Pixel Value (U8, U16, I16, Float)"=sgl 255.0, "Image Mask"=w377, "Image"=w377) -> ("error out"=w370:errorcluster, "Image Out"=w371:T2)  [unwired: 6 in]
        n257 = Wait (ms)(milliseconds to wait=u32 50 ("等待时间（毫秒）")) -> ()  [unwired: 1 out]
        n258 = call "IMAQ AutoBThreshold 2"("Image Src"=w371, "Look For (Bright Objects)"=w374, "Method (clustering)"=w373, "Image Dst"=w365, "error in (no error)"=w370, "Threshold Limits"=cluster{"Lower value":sgl, "Upper value":sgl} {"Lower value"=1.0, "Upper value"=255.0}) -> ("Image Dst Out"=w368:T2)  [unwired: 2 in, 7 out]
        n259 = call "IMAQ FillHole"("Image Dst"=w365, "Image Src"=w368, "Connectivity 4/8 (8)"=TRUE) -> ("Image Dst Out"=w366:T2)  [unwired: 3 in, 1 out]
        n260 = call "IMAQ RemoveParticle"("Number of Erosion"=12, "Image Dst"=w365, "Image Src"=w366) -> ("Image Dst Out"=w358:T2)  [unwired: 7 in, 1 out]
        n261 = call "IMAQ MaskToROI"("Image"=w358, "Max number of vectors in ROI"=50000) -> ("ROI Descriptor"=w355:T8)  [unwired: 5 in, 2 out]
        n262 = call "IMAQ Overlay ROI"("ROI Descriptor"=w355, "Image"=w358) -> ("Image Out"=w354:T2)  [unwired: 8 in, 1 out]
        n263 = call "IMAQ Overlay ROI"("ROI Descriptor"=w355, "Image"=w357) -> ("Image Out"=w356:T2)  [unwired: 8 in, 1 out]
        n264 = local write "单幅画面"(w354) -> ()
        n265 = local write "Threshold Image"(w356) -> ()
        n266 = local read "叠加画面"() -> (w390:T2)
        n267 = local read "总像素"() -> (w391:dbl)
      }
    }
    n268 = Merge Errors(w169, w171, w170) -> (w178:errorcluster)
    n269 = Compound Arithmetic op=OR ("复合运算")(w178, "Stop") -> (w180:bool)
  }
  n270 = call "IMAQ Dispose"("Image"=w18) -> ("error out"=w34:errorcluster)  [unwired: 2 in, 3 out]
  n271 = call <vilib>:"Simple Error Handler.vi"("error in (no error)"=w34) -> ()  [unwired: 1 in, 8 out]
  n272 = call <vilib>:"Simple Error Handler.vi"("error in (no error)"=w5) -> ()  [unwired: 1 in, 8 out]
  n273 = stacked-sequence {
    seq-local: [_ w397 _] -> [_ _ w403]
    tunnel: w28 -> [_ _ w402]
    tunnel: w14 -> [_ _ w401]
    frame #0 {
      n274 = disable-structure shown="禁用" {
        frame Disabled {
          n275 = Two Button Dialog(message="火焰分割已结束，是否回看" ("消息"), 1:"否" ("F按钮名称（“取消”）"), 2:"是" ("T按钮名称（“确定”）")) -> (T button?=w393:bool)
          n276 = case shown="真" w393 {
            frame False {
            }
            frame True {
              n277 = call "单帧回看.vi"() -> ()  [unwired: 28 in]
            }
          }
        }
        frame Enabled {
        }
      }
    }
    frame #1 {
      n278 = Two Button Dialog(message="是否要进行手动操作，消除地面的影响" ("消息")) -> (T button?=w397:bool)  [unwired: 2 in]
    }
    frame #2 {
      n279 = case shown="真" w403 {
        tunnel: w402 -> [_ w405]
        tunnel: w401 -> [_ w404]
        frame False {
        }
        frame True {
          n280 = call "handclear.vi"("总像素"=w404, "Image 3"=w405) -> ()  [unwired: 10 in]
        }
      }
      n281 = property on="返回主界面" class="Bool (严格)"("DisabledEnum"=T3."Enabled" ("禁用")) -> ()  [unwired: 2 in, 2 out]
      n282 = property on="保存" class="Bool (严格)"("DisabledEnum"=T3."Enabled" ("禁用")) -> ()  [unwired: 2 in, 2 out]
    }
  }
  "导入像素当量" <- FALSE ("导入像素当量")
